vi "Array Panel Async.vi"(10 "Container":refnum<vi>, 11 "2DArrayManager":refnum<class "2DArrayManager.lvclass">) -> ()   [LabVIEW 2020, in "OOPanel.lvlib" / "2DArrayManager.lvclass"]
uses:
  2DArrayManager.lvclass
  2DArrayManager.lvclass/2DArrayManager.ctl
panel:
  in  "Corner":bool
  in  "VBar":i32(c297)
  in  "HBar":i32(c297)
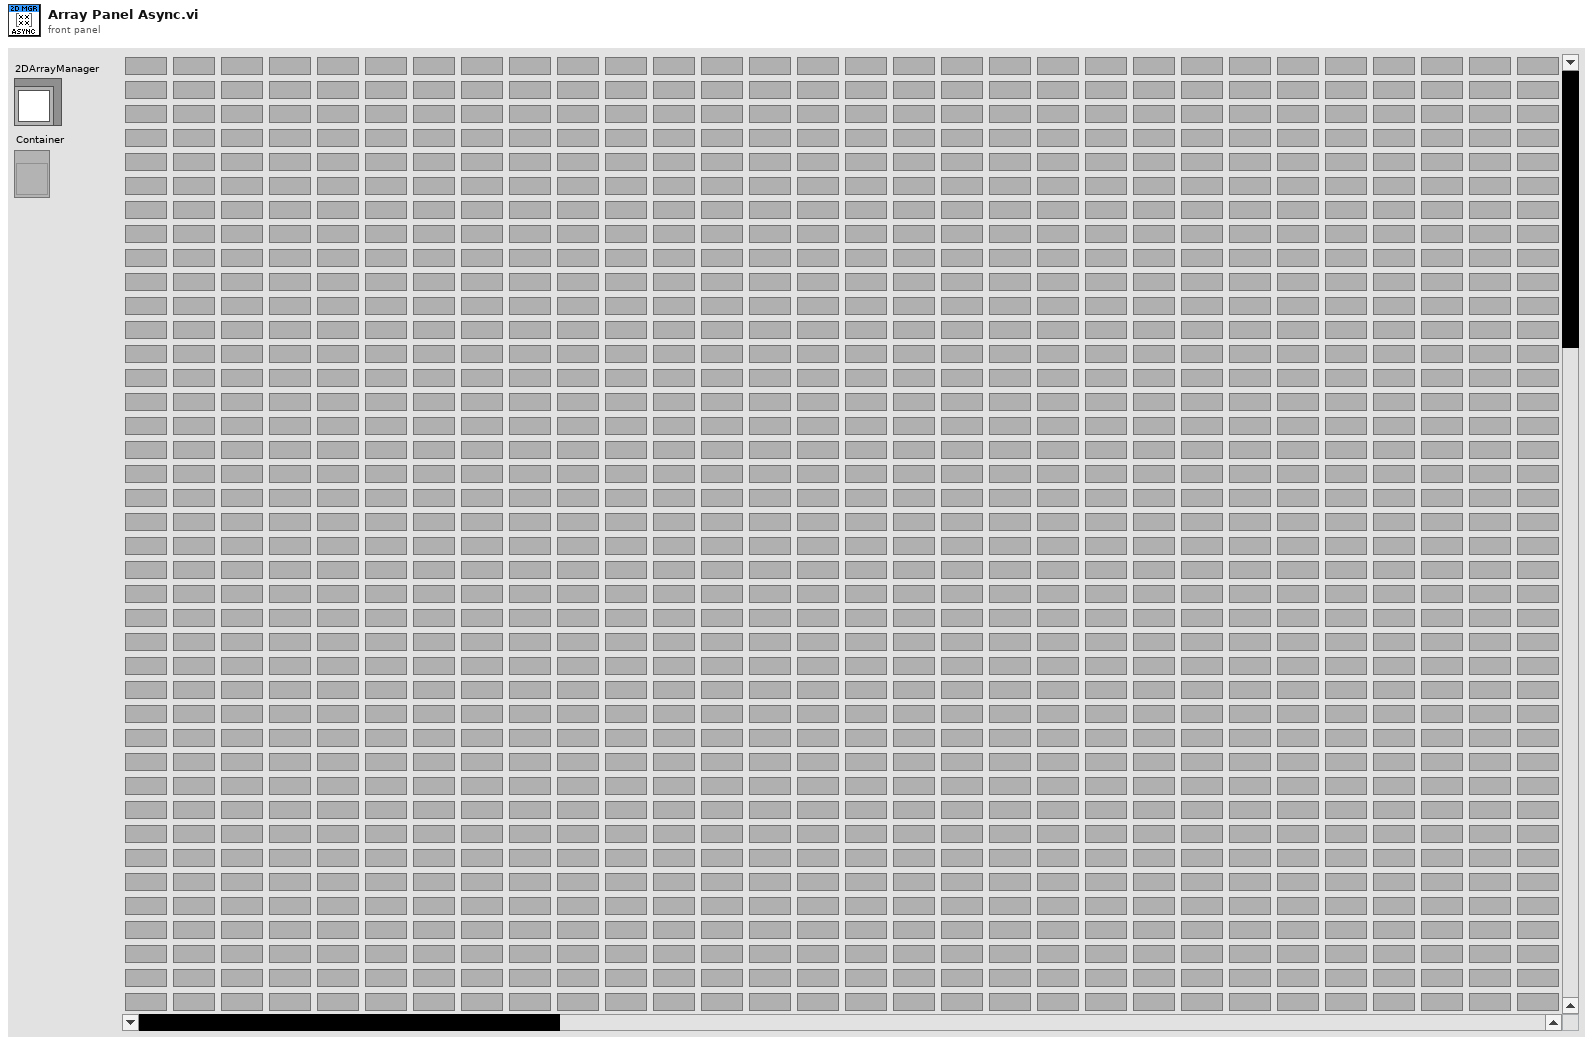
[diagram p1: front panel]
types:
  T1 = typedef "OOPanel.lvlib/2DArrayManager.lvclass/Direction.ctl" = enum16{"Vertical", "Horizontal", "Both"}
  T2 = typedef "OOPanel.lvlib/2DArrayManager.lvclass/Options.ctl" = cluster{"Running":bool, "Borders":bool, "Background":u32, "V Scroll":bool, "H Scroll":bool}
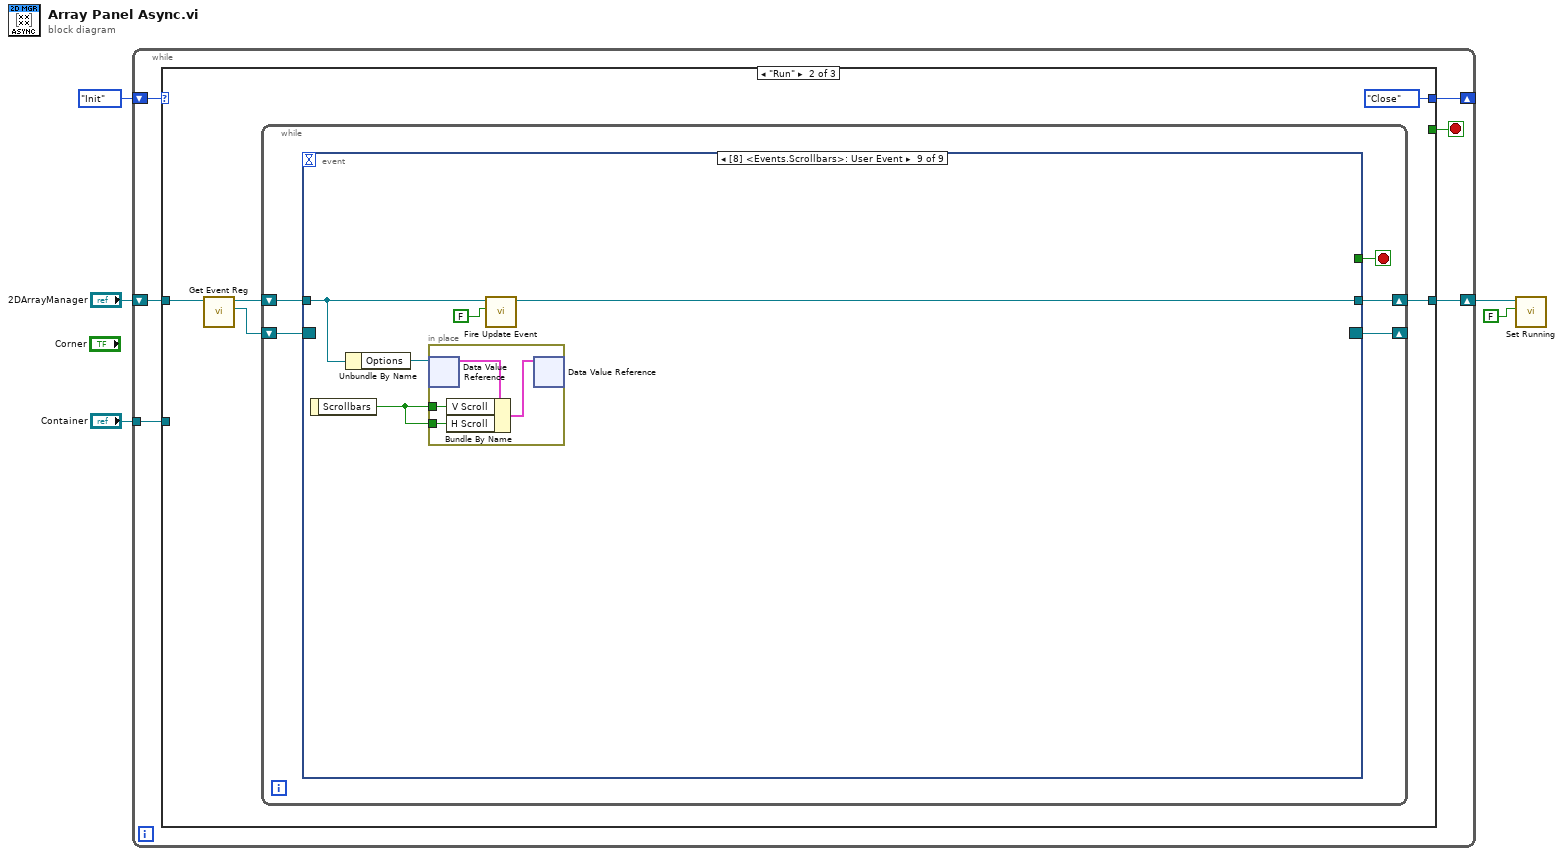
[diagram p0: block diagram]
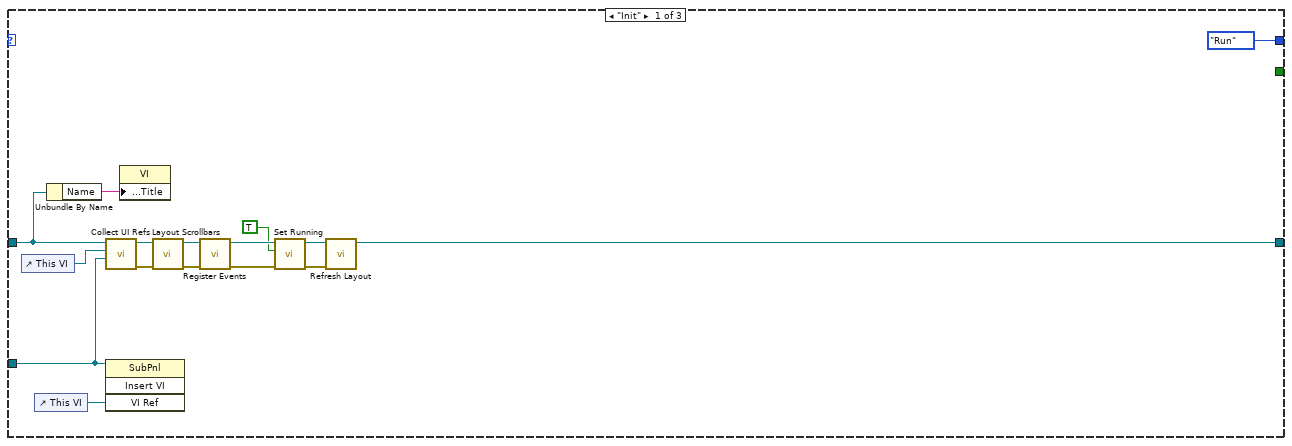
[diagram p2: hidden frame]
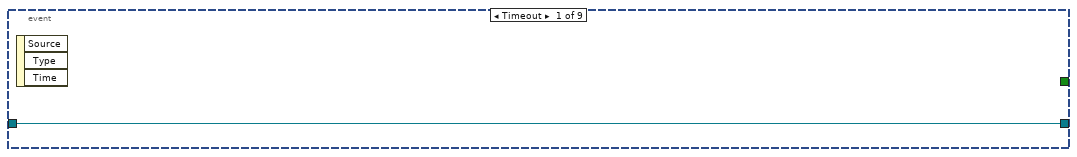
[diagram p3: hidden frame]
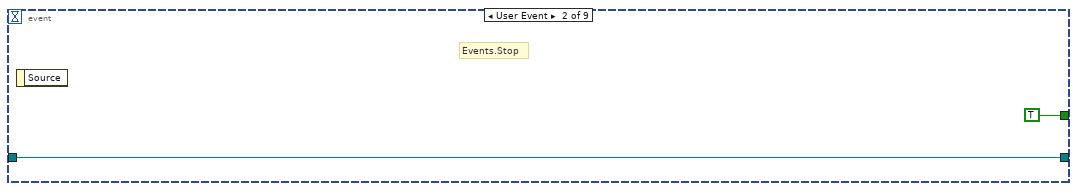
[diagram p4: hidden frame]
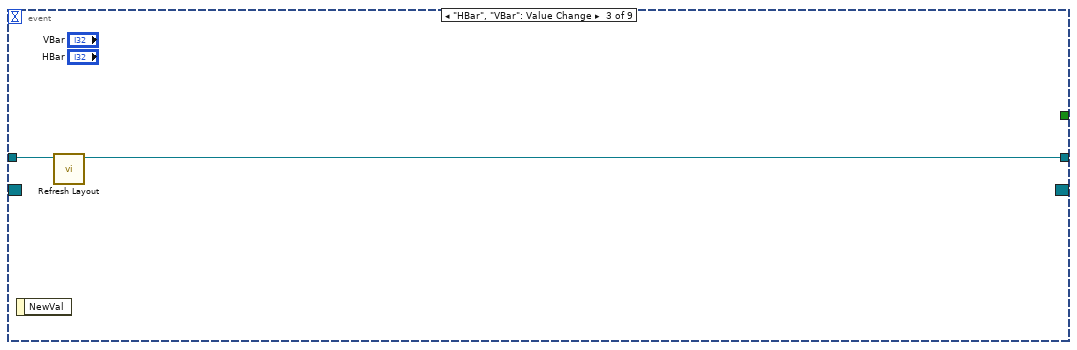
[diagram p5: hidden frame]
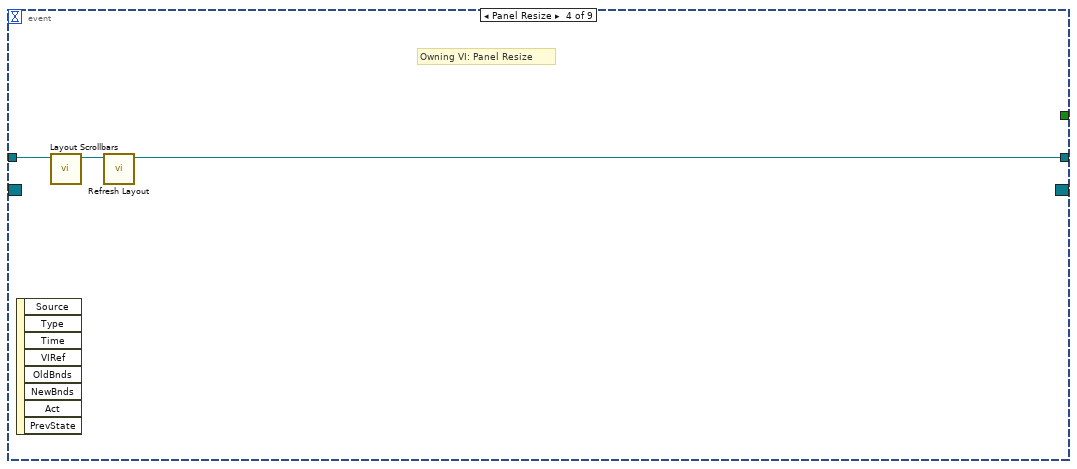
[diagram p6: hidden frame]
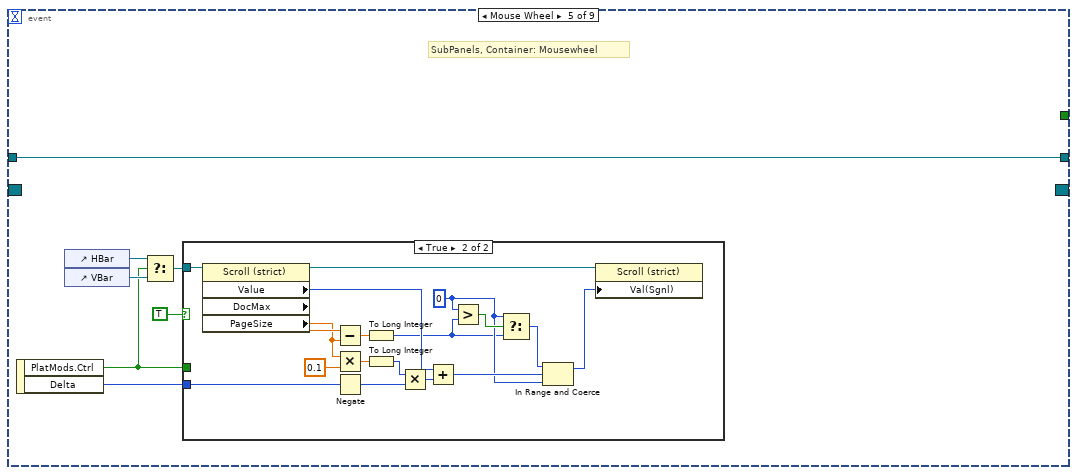
[diagram p7: hidden frame]
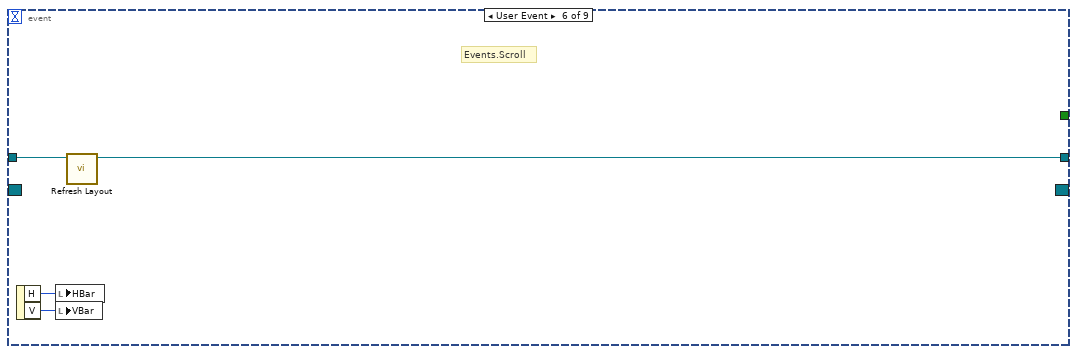
[diagram p9: hidden frame]
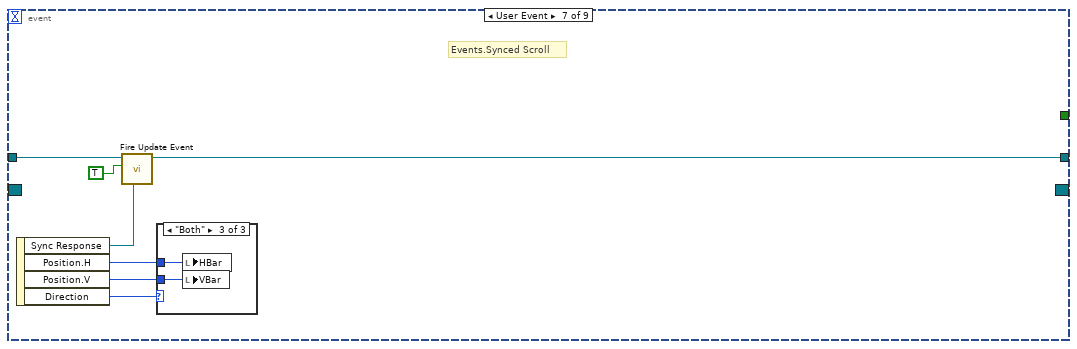
[diagram p10: hidden frame]
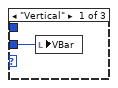
[diagram p11: hidden frame]
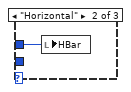
[diagram p12: hidden frame]
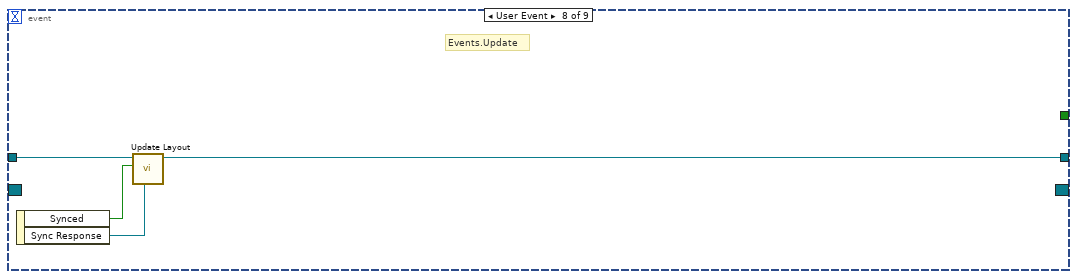
[diagram p13: hidden frame]
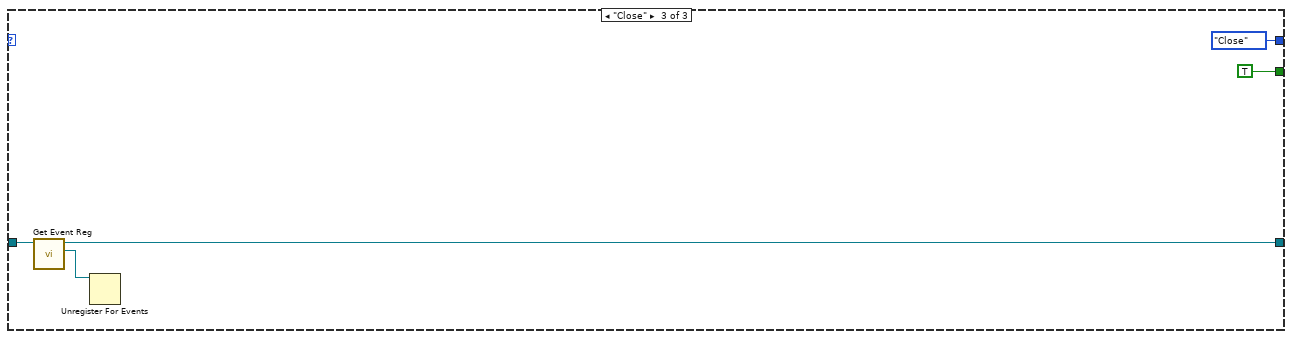
[diagram p14: hidden frame]
diagram:
  n1 = while {
    shift-right: [w10] -> _
    shift-left: enum16{"Init", "Run", "Close"}."Init" -> [w11]
    shift-right: [w7] -> w2
    shift-left: "2DArrayManager" -> [w9]
    tunnel: "Container" -> [w8]
    stop <- w6 stop-if-true
    n2 = case shown="\"Run\"" w11 {
      tunnel: [enum16{"Init", "Run", "Close"}."Run" enum16{"Init", "Run", "Close"}."Close" enum16{"Init", "Run", "Close"}."Close"] -> w10
      tunnel: w9 -> [w24 w31 w101]
      tunnel: w8 -> [w12 _ _]
      tunnel: [w15 w28 w100] -> w7
      tunnel: [_ _ TRUE] -> w6
      frame "Init" {
        n3 = control-ref of="This VI"() -> (w25:refnum<vi>)
        n4 = control-ref of="This VI"() -> (w26:refnum<vi>)
        n5 = Unbundle By Name(w24) -> ("Name"=w23:string)
        n6 = call "Collect UI Refs.vi"("Container"=w12, "Layout Panel VI"=w25, "2DArrayManager in"=w24) -> ("error out"=w21:errorcluster, "2DArrayManager out"=w22:refnum<class "2DArrayManager.lvclass">)  [unwired: 7 in]
        n7 = invoke class="SubPnl" method="Insert VI"(reference=w12, "VI Ref"=w26) -> ()  [unwired: 2 in, 4 out]
        n8 = property class="VI"("Front Panel.Title"=w23) -> ()  [unwired: 2 in, 2 out]
        n9 = call "Layout Scrollbars.vi"("error in (no error)"=w21, "2DArrayManager in"=w22) -> ("error out"=w19:errorcluster, "2DArrayManager out"=w20:refnum<class "2DArrayManager.lvclass">)  [unwired: 8 in]
        n10 = call "Register Events.vi"("error in (no error)"=w19, "2DArrayManager in"=w20) -> ("error out"=w13:errorcluster, "2DArrayManager out"=w18:refnum<class "2DArrayManager.lvclass">)  [unwired: 8 in]
        n11 = call "Set Running.vi"("error in (no error)"=w13, "Running"=TRUE, "2DArrayManager in"=w18) -> ("error out"=w14:errorcluster, "2DArrayManager out"=w17:refnum<class "2DArrayManager.lvclass">)  [unwired: 7 in]
        n12 = call "Refresh Layout.vi"("error in (no error)"=w14, "2DArrayManager in"=w17) -> ("2DArrayManager out"=w15:refnum<class "2DArrayManager.lvclass">)  [unwired: 8 in, 1 out]
      }
      frame "Run" {
        n13 = call "Get Event Reg.vi"("2DArrayManager in"=w31) -> ("Event Reg"=w29:refnum<event-registration>, "2DArrayManager out"=w30:refnum<class "2DArrayManager.lvclass">)  [unwired: 8 in, 1 out]
        n14 = while {
          shift-right: [w37] -> w28
          shift-left: w30 -> [w36]
          shift-right: [w35] -> _
          shift-left: w29 -> [w33]
          stop <- w34 stop-if-true
          n15 = event shown="[8] <Events.Scrollbars>: User Event" {
            selector: w33 -> [_ _ _ _ _ _ _ _ _]
            dyn-events: [_ _ _ _ _ _ _ _ _] -> w35
            timeout: _ -> [_ _ _ _ _ _ _ _ _]
            tunnel: [w38 w40 w41 w43 w52 w71 w77 w88 w91] -> w37
            tunnel: w36 -> [w38 w40 w42 w45 w52 w74 w78 w89 w93]
            tunnel: [_ TRUE _ _ _ _ _ _ _] -> w34
            event Timeout {
              n16 = event-data() -> ()  [unwired: 1 in, 3 out]
            }
            event User Event {
              # "Events.Stop"
              n17 = event-data() -> ()  [unwired: 1 in, 1 out]
            }
            event "HBar", "VBar": Value Change {
              n18 = event-data() -> ()  [unwired: 1 in, 1 out]
              n19 = call "Refresh Layout.vi"("2DArrayManager in"=w42) -> ("2DArrayManager out"=w41:refnum<class "2DArrayManager.lvclass">)  [unwired: 9 in, 1 out]
            }
            event Panel Resize {
              # "Owning VI: Panel Resize"
              n20 = event-data() -> ()  [unwired: 1 in, 8 out]
              n21 = call "Layout Scrollbars.vi"("2DArrayManager in"=w45) -> ("2DArrayManager out"=w44:refnum<class "2DArrayManager.lvclass">)  [unwired: 9 in, 1 out]
              n22 = call "Refresh Layout.vi"("2DArrayManager in"=w44) -> ("2DArrayManager out"=w43:refnum<class "2DArrayManager.lvclass">)  [unwired: 9 in, 1 out]
            }
            event Mouse Wheel {
              # "SubPanels, Container: Mousewheel"
              n23 = event-data() -> ("PlatMods.Ctrl"=w46:bool, "Delta"=w48:i32)  [unwired: 1 in]
              n24 = control-ref of="HBar"() -> (w51:refnum<vi>)
              n25 = control-ref of="VBar"() -> (w50:refnum<vi>)
              n26 = Select(t=w51, s=w46, f=w50) -> (s? t:f=w49:refnum<vi>)
              n27 = case shown="True" TRUE {
                tunnel: w48 -> [_ w53]
                tunnel: w49 -> [_ w55]
                tunnel: w46 -> [_ _]
                frame False {
                }
                frame True {
                  w58 = 0 ("lower limit")
                  n28 = property on="Property Node" class="Scroll (strict)"(reference=w55) -> (reference out=w54:refnum<vi>, "Value"=w66:i32, "DocMax"=w64:dbl, "PageSize"=w63:dbl)  [unwired: 1 in, 1 out]
                  n29 = Subtract(x=w64, y=w63) -> (x-y=w62:dbl)
                  n30 = Multiply(x=w63, y=0.1) -> (x*y=w69:dbl)
                  n31 = Negate(x=w53) -> (-x=w60:i32)
                  n32 = To Long Integer(number=w62) -> (32bit integer=w57:i32)
                  n33 = To Long Integer(number=w69) -> (32bit integer=w67:i32)
                  n34 = Multiply(x=w67, y=w60) -> (x*y=w68:i32)
                  n35 = Add(x=w66, y=w68) -> (x+y=w65:i32)
                  n36 = Greater?(x=w58, y=w57) -> (0:w59:bool)
                  n37 = Select(t=w58, s=w59, f=w57) -> (s? t:f=w56:i32)
                  n38 = In Range and Coerce(upper limit=w56, x=w65, lower limit=w58) -> (coerced(x)=w61:i32)  [unwired: 1 out]
                  n39 = property on="Property Node" class="Scroll (strict)"(reference=w54, "Val(Sgnl)"=w61) -> ()  [unwired: 1 in, 2 out]
                }
              }
            }
            event User Event {
              # "Events.Scroll"
              n40 = event-data() -> ("H"=w73:i32, "V"=w72:i32)  [unwired: 1 in]
              n41 = local write "HBar"(w73) -> ()
              n42 = local write "VBar"(w72) -> ()
              n43 = call "Refresh Layout.vi"("2DArrayManager in"=w74) -> ("2DArrayManager out"=w71:refnum<class "2DArrayManager.lvclass">)  [unwired: 9 in, 1 out]
            }
            event User Event {
              # "Events.Synced Scroll"
              n44 = event-data() -> ("Sync Response"=w75:refnum<notifier>, "Position.H"=w81:i32, "Position.V"=w80:i32, "Direction"=w79:T1)  [unwired: 1 in]
              n45 = call "Fire Update Event.vi"("Sync Response"=w75, "Synced"=TRUE, "2DArrayManager in"=w78) -> ("2DArrayManager out"=w77:refnum<class "2DArrayManager.lvclass">)  [unwired: 7 in, 1 out]
              n46 = case shown="\"Both\"" w79 {
                tunnel: w81 -> [_ w83 w85]
                tunnel: w80 -> [w82 _ w84]
                frame "Vertical" {
                  n47 = local write "VBar"(w82) -> ()
                }
                frame "Horizontal" {
                  n48 = local write "HBar"(w83) -> ()
                }
                frame "Both" {
                  n49 = local write "HBar"(w85) -> ()
                  n50 = local write "VBar"(w84) -> ()
                }
              }
            }
            event User Event {
              # "Events.Update"
              n51 = event-data() -> ("Synced"=w87:bool, "Sync Response"=w86:refnum<notifier>)  [unwired: 1 in]
              n52 = call "Update Layout.vi"("Sync Response"=w86, "Synced"=w87, "2DArrayManager in"=w89) -> ("2DArrayManager out"=w88:refnum<class "2DArrayManager.lvclass">)  [unwired: 7 in, 1 out]
            }
            event User Event {
              n53 = event-data() -> ("Scrollbars"=w92:bool)  [unwired: 1 in]
              n54 = Unbundle By Name(w93) -> ("Options"=w94:refnum<data-value>)
              n55 = in-place {
                in-place-border: w92 -> [w96]
                in-place-border: w92 -> [w95]
                n56 = in-place-dvr #1(w94) -> (w98:T2)  [unwired: 1 out]
                n57 = Bundle By Name(cluster=w98, "V Scroll"=w96, "H Scroll"=w95) -> (w97:T2)
                n58 = in-place-dvr #1(w97) -> ()  [unwired: 2 out]
              }
              n59 = call "Fire Update Event.vi"("Synced"=FALSE, "2DArrayManager in"=w93) -> ("2DArrayManager out"=w91:refnum<class "2DArrayManager.lvclass">)  [unwired: 8 in, 1 out]
            }
          }
        }
      }
      frame "Close" {
        n60 = call "Get Event Reg.vi"("2DArrayManager in"=w101) -> ("Event Reg"=w99:refnum<event-registration>, "2DArrayManager out"=w100:refnum<class "2DArrayManager.lvclass">)  [unwired: 8 in, 1 out]
        n61 = Unregister For Events(event registration refnum=w99) -> ()  [unwired: 1 in, 1 out]
      }
    }
  }
  n62 = call "Set Running.vi"("Running"=FALSE, "2DArrayManager in"=w2) -> ()  [unwired: 8 in, 2 out]
